vi "MB setzen.vi"(10 "Def.CalGas Alt":T1 {"Messbereiche"."Messbereich 12" items=["0-100ppm", "0-1000ppm", "0-5000ppm"]; "Messbereiche"."Messbereich 11" items=["0-100ppm", "0-1000ppm", "0-5000ppm"]; "Messbereiche"."Messbereich 10" items=["0-100ppm", "0-1000ppm", "0-5000ppm"]; "Messbereiche"."Messbereich 9" items=["0-100ppm", "0-1000ppm", "0-5000ppm"]; "Messbereiche"."Messbereich 8" items=["0-100ppm", "0-1000ppm", "0-5000ppm"]; "Messbereiche"."Messbereich 7" items=["0-100ppm", "0-1000ppm", "0-5000ppm"]; "Messbereiche"."Messbereich 6" items=["0-100ppm", "0-1000ppm", "0-5000ppm"]; "Messbereiche"."Messbereich 5" items=["0-100ppm", "0-1000ppm", "0-5000ppm"]; "Messbereiche"."Messbereich 4" items=["0-100ppm", "0-1000ppm", "0-5000ppm"]; "Messbereiche"."Messbereich 3" items=["0-100ppm", "0-1000ppm", "0-5000ppm"]; "Messbereiche"."Messbereich 2" items=["0-100ppm", "0-1000ppm", "0-5000ppm"]; "Messbereiche"."Messbereich 1" items=["0-100ppm", "0-1000ppm", "0-5000ppm"]; "Einheit"."Einheit 12" items=["ppm", "%"]; "Einheit"."Einheit 11" items=["ppm", "%"]; "Einheit"."Einheit 10" items=["ppm", "%"]; "Einheit"."Einheit 9" items=["ppm", "%"]; "Einheit"."Einheit 8" items=["ppm", "%"]; "Einheit"."Einheit 7" items=["ppm", "%"]; "Einheit"."Einheit 6" items=["ppm", "%"]; "Einheit"."Einheit 5" items=["ppm", "%"]; "Einheit"."Einheit 4" items=["ppm", "%"]; "Einheit"."Einheit 3" items=["ppm", "%"]; "Einheit"."Einheit 2" items=["ppm", "%"]; "Einheit"."Einheit 1" items=["ppm", "%"]; "Werte 2"."Konzentration 12" format="%#_5g"; "Werte 2"."Konzentration 11" format="%#_5g"; "Werte 2"."Konzentration 10" format="%#_5g"; "Werte 2"."Konzentration 9" format="%#_5g"; "Werte 2"."Konzentration 8" format="%#_5g"; "Werte 2"."Konzentration 7" format="%#_5g"; "Werte 2"."Konzentration 6" format="%#_5g"; "Werte 2"."Konzentration 5" format="%#_5g"; "Werte 2"."Konzentration 4" format="%#_5g"; "Werte 2"."Konzentration 3" format="%#_5g"; "Werte 2"."Konzentration 2" format="%#_5g"; "Werte 2"."Konzentration 1" format="%#_5g"; "Werte"."Konzentration 12" format="%#_5g"; "Werte"."Konzentration 11" format="%#_5g"; "Werte"."Konzentration 10" format="%#_5g"; "Werte"."Konzentration 9" format="%#_5g"; "Werte"."Konzentration 8" format="%#_5g"; "Werte"."Konzentration 7" format="%#_5g"; "Werte"."Konzentration 6" format="%#_5g"; "Werte"."Konzentration 5" format="%#_5g"; "Werte"."Konzentration 4" format="%#_5g"; "Werte"."Konzentration 3" format="%#_5g"; "Werte"."Konzentration 2" format="%#_5g"; "Werte"."Konzentration 1" format="%#_5g"}, 11 "Def.CalGas Neu":T1 {"Messbereiche"."Messbereich 12" items=["0-100ppm", "0-1000ppm", "0-5000ppm"]; "Messbereiche"."Messbereich 11" items=["0-100ppm", "0-1000ppm", "0-5000ppm"]; "Messbereiche"."Messbereich 10" items=["0-100ppm", "0-1000ppm", "0-5000ppm"]; "Messbereiche"."Messbereich 9" items=["0-100ppm", "0-1000ppm", "0-5000ppm"]; "Messbereiche"."Messbereich 8" items=["0-100ppm", "0-1000ppm", "0-5000ppm"]; "Messbereiche"."Messbereich 7" items=["0-100ppm", "0-1000ppm", "0-5000ppm"]; "Messbereiche"."Messbereich 6" items=["0-100ppm", "0-1000ppm", "0-5000ppm"]; "Messbereiche"."Messbereich 5" items=["0-100ppm", "0-1000ppm", "0-5000ppm"]; "Messbereiche"."Messbereich 4" items=["0-100ppm", "0-1000ppm", "0-5000ppm"]; "Messbereiche"."Messbereich 3" items=["0-100ppm", "0-1000ppm", "0-5000ppm"]; "Messbereiche"."Messbereich 2" items=["0-100ppm", "0-1000ppm", "0-5000ppm"]; "Messbereiche"."Messbereich 1" items=["0-100ppm", "0-1000ppm", "0-5000ppm"]; "Einheit"."Einheit 12" items=["ppm", "%"]; "Einheit"."Einheit 11" items=["ppm", "%"]; "Einheit"."Einheit 10" items=["ppm", "%"]; "Einheit"."Einheit 9" items=["ppm", "%"]; "Einheit"."Einheit 8" items=["ppm", "%"]; "Einheit"."Einheit 7" items=["ppm", "%"]; "Einheit"."Einheit 6" items=["ppm", "%"]; "Einheit"."Einheit 5" items=["ppm", "%"]; "Einheit"."Einheit 4" items=["ppm", "%"]; "Einheit"."Einheit 3" items=["ppm", "%"]; "Einheit"."Einheit 2" items=["ppm", "%"]; "Einheit"."Einheit 1" items=["ppm", "%"]; "Werte 2"."Konzentration 12" format="%#_5g"; "Werte 2"."Konzentration 11" format="%#_5g"; "Werte 2"."Konzentration 10" format="%#_5g"; "Werte 2"."Konzentration 9" format="%#_5g"; "Werte 2"."Konzentration 8" format="%#_5g"; "Werte 2"."Konzentration 7" format="%#_5g"; "Werte 2"."Konzentration 6" format="%#_5g"; "Werte 2"."Konzentration 5" format="%#_5g"; "Werte 2"."Konzentration 4" format="%#_5g"; "Werte 2"."Konzentration 3" format="%#_5g"; "Werte 2"."Konzentration 2" format="%#_5g"; "Werte 2"."Konzentration 1" format="%#_5g"; "Werte"."Konzentration 12" format="%#_5g"; "Werte"."Konzentration 11" format="%#_5g"; "Werte"."Konzentration 10" format="%#_5g"; "Werte"."Konzentration 9" format="%#_5g"; "Werte"."Konzentration 8" format="%#_5g"; "Werte"."Konzentration 7" format="%#_5g"; "Werte"."Konzentration 6" format="%#_5g"; "Werte"."Konzentration 5" format="%#_5g"; "Werte"."Konzentration 4" format="%#_5g"; "Werte"."Konzentration 3" format="%#_5g"; "Werte"."Konzentration 2" format="%#_5g"; "Werte"."Konzentration 1" format="%#_5g"}) -> ()   [LabVIEW 2020, in "CalGas Aufschaltung.lvlib"]
uses:
  CalGas Aufschaltung.lvlib
  Definition CalGas Anzeige.ctl
  CalGas-Namen.ctl
  Visualisierungs Elemente/String - Eingabefeld.ctl
  CalGas-Werte.ctl
  Visualisierungs Elemente/Zahlen-Eingabefeld.ctl
  CalGas-Einheit.ctl
  Visualisierungs Elemente/Auswahlfeld.ctl
  CalGas-Messbereiche.ctl
  Analysator Definition/FGV Analysator Definition Aktionen.ctl
  Analysator Definition/Analysator Definition.lvlib
  Messdaten/Messdaten.lvlib
panel:
  # "Span 1"
  # "Span 2"
  # "Span 3"
  # "Span 4"
  # "Span 5"
  # "Span 6"
  # "Span 7"
  # "Span 8"
  # "Span 9"
  # "Span 10"
  # "Span 11"
  # "Span 12"
  # "Span 1"
  # "Span 2"
  # "Span 3"
  # "Span 4"
  # "Span 5"
  # "Span 6"
  # "Span 7"
  # "Span 8"
  # "Span 9"
  # "Span 10"
  # "Span 11"
  # "Span 12"
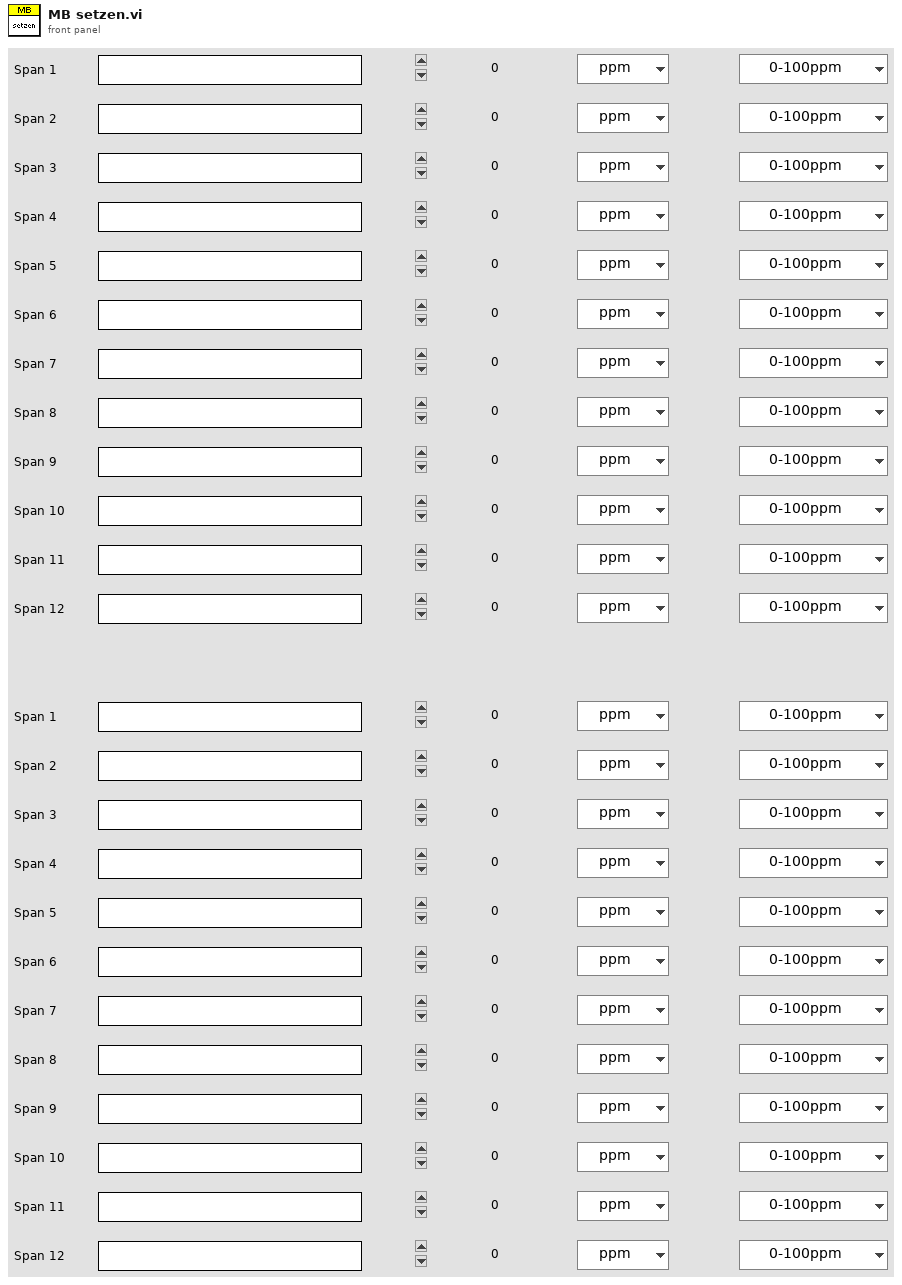
[diagram p1: front panel]
types:
  T1 = typedef "CalGas Aufschaltung.lvlib/Definition CalGas Anzeige.ctl" = cluster{"Namen":T2, "Werte":T4, "Werte 2":T4, "Einheit":T6, "Messbereiche":T8}
  T2 = typedef "CalGas Aufschaltung.lvlib/CalGas-Namen.ctl" = cluster{"Name":T3, "Name 2":T3, "Name 3":T3, "Name 4":T3, "Name 5":T3, "Name 6":T3, "Name 7":T3, "Name 8":T3, "Name 9":T3, "Name 10":T3, "Name 11":T3, "Name 12":T3}
  T3 = typedef "String - Eingabefeld.ctl" = string
  T4 = typedef "CalGas Aufschaltung.lvlib/CalGas-Werte.ctl" = cluster{"Konzentration 1":T5, "Konzentration 2":T5, "Konzentration 3":T5, "Konzentration 4":T5, "Konzentration 5":T5, "Konzentration 6":T5, "Konzentration 7":T5, "Konzentration 8":T5, "Konzentration 9":T5, "Konzentration 10":T5, "Konzentration 11":T5, "Konzentration 12":T5}
  T5 = typedef "Zahlen-Eingabefeld.ctl" = sgl
  T6 = typedef "CalGas Aufschaltung.lvlib/CalGas-Einheit.ctl" = cluster{"Einheit 1":T7, "Einheit 2":T7, "Einheit 3":T7, "Einheit 4":T7, "Einheit 5":T7, "Einheit 6":T7, "Einheit 7":T7, "Einheit 8":T7, "Einheit 9":T7, "Einheit 10":T7, "Einheit 11":T7, "Einheit 12":T7}
  T7 = typedef "Auswahlfeld.ctl" = u16
  T8 = typedef "CalGas Aufschaltung.lvlib/CalGas-Messbereiche.ctl" = cluster{"Messbereich 1":T7, "Messbereich 2":T7, "Messbereich 3":T7, "Messbereich 4":T7, "Messbereich 5":T7, "Messbereich 6":T7, "Messbereich 7":T7, "Messbereich 8":T7, "Messbereich 9":T7, "Messbereich 10":T7, "Messbereich 11":T7, "Messbereich 12":T7}
  T9 = typedef "Analysator Definition.lvlib/FGV Analysator Definition Aktionen.ctl" = enum16{"lesen", "MB setzen", "MB KAL setzen", "laden"}
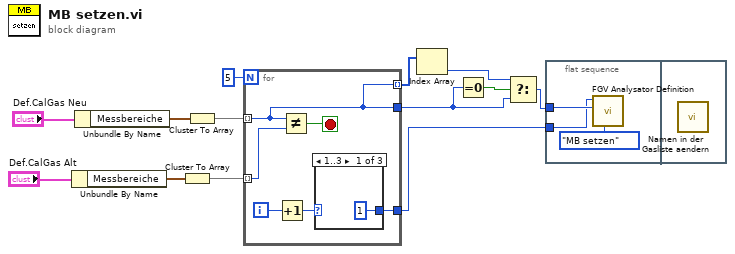
[diagram p0: block diagram]
diagram:
  n1 = Unbundle By Name("Def.CalGas Alt") -> ("Messbereiche"=w10:T8)
  n2 = Unbundle By Name("Def.CalGas Neu") -> ("Messbereiche"=w11:T8)
  n3 = Cluster To Array(cluster=w10) -> (array=w8:T7[])
  n4 = Cluster To Array(cluster=w11) -> (array=w9:T7[])
  n5 = for {
    N: 5 -> [_]
    tunnel: w9 -> [w15] mode=indexing
    tunnel: w8 -> [w19] mode=indexing
    tunnel: [w15] -> w4
    tunnel: [w16] -> w7
    tunnel: [w15] -> w2 mode=indexing
    i -> [w14]
    stop <- w18 stop-if-true
    n6 = Increment(x=w14) -> (x+1=w17:i32)
    n7 = Not Equal?(x=w15, y=w19) -> (x != y?=w18:bool)
    n8 = case shown="1..3" w17 {
      selector: w17 -> [_ w21 w22]
      tunnel: [1 w21 w22] -> w16
      frame 1..3 {
      }
      frame 0, Default {
      }
      frame 5..7 {
      }
    }
  }
  n9 = Index Array(array=w2) -> (element=w1:T7)  [unwired: 1 in]
  n10 = Equal To 0?(x=w4) -> (x = 0?=w5:bool)
  n11 = Select(t=w1, s=w5, f=w4) -> (s? t:f=w3:T7)
  n12 = flat-sequence {
    tunnel: w3 -> [w24]
    tunnel: w7 -> [w23]
    frame #0 {
      n13 = call "FGV Analysator Definition.vi"("Aktionen"=FGV_Analysator_Definition_Aktionen."MB setzen", "Messbereich"=w24, "Komponente"=w23) -> ()  [unwired: 4 in, 5 out]
    }
    frame #1 {
      n14 = call "Namen in der Gasliste aendern.vi"() -> ()  [unwired: 12 in]
    }
  }
